vi "ALTS-2015 Confirm Test Selection DI.vi"(8 "error in":errorcluster, 11 "Station Cluster":T1) -> (0 "error out":errorcluster, 3 "Test Type Selection Successful":bool)   [LabVIEW 2013]
uses:
  Controls/ALTS-2015 Station Cluster.ctl
  Controls/ALTS-2015 LV2GBL Station Info Options.ctl
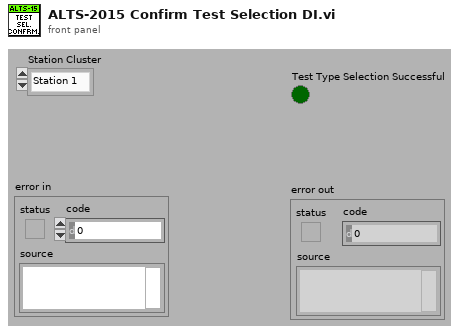
[diagram p1: front panel]
types:
  T1 = typedef "ALTS-2015 Station Cluster.ctl" = enum16{"Station 1", "Station 2", "Station 3", "Station 4"}
  T2 = typedef "ALTS-2015 LV2GBL Station Info Options.ctl" = enum16{"Init", "Read", "Read All", "Write Sensor ID", "Write  Work Order", "Write Serial Number", "Write Test Data", "Write Station Status", "Write Station Occupancy", "Write Station Test Type", "Write Rerun", "Write Load Decision", "Write Robot Action", "Clear All", "Clear Test Result"}
  T3 = typedef "ALTS-2015 Station Details.ctl" = cluster{"Station Number":string, "Work Order Number":string, "Sensor Name":string, "Pressure (PSI)":string, "Flow (SCCM)":string, "Test Time ":string, "Test Result":string, "Serial Number":string, "Station Status":T4, "SW assigned UUT":bool, "Rerun Count":i32, "Test Type":i32, "Load Decision":i32, "Robot Action":T5}
  T4 = typedef "ALTS-2015 Status Ring Indicator.ctl" = u16
  T5 = typedef "ALTS-2015 Robot Actions.ctl" = enum16{"Loading...", "Unloading...", "Reruning...", "No Action"}
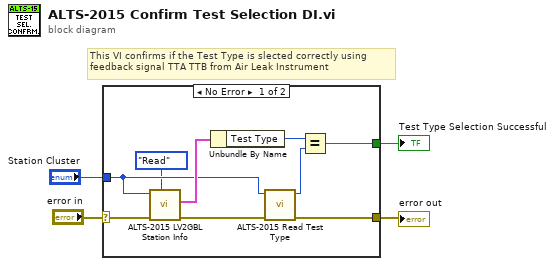
[diagram p0: block diagram]
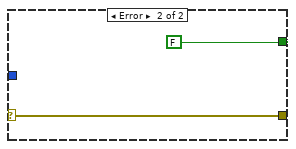
[diagram p2: hidden frame]
diagram:
  # "This VI confirms if the Test Type is slected correctly using \nfeedback signal TTA TTB from Air Leak Instrument"
  n1 = case shown="No Error" "error in" {
    selector: "error in" -> [w13 w15]
    tunnel: [w12 w15] -> w4
    tunnel: "Station Cluster" -> [w9 _]
    tunnel: [w7 FALSE] -> w1
    frame No Error {
      n2 = call "ALTS-2015 LV2GBL Station Info.vi"("Options"=ALTS-2015_LV2GBL_Station_Info_Options."Read", "error in"=w13, "Station Cluster"=w9) -> ("error out"=w11:errorcluster, "Station Details"=w10:T3)  [unwired: 6 in, 1 out]
      n3 = Unbundle By Name(w10) -> ("Test Type"=w8:i32)
      n4 = call "ALTS-2015 Read Test Type.vi"("error in"=w11, "Station Cluster"=w9) -> ("error out"=w12:errorcluster, "Test Type"=w6:i32)  [unwired: 8 in]
      n5 = Equal?(x=w8, y=w6) -> (x = y?=w7:bool)
    }
    frame Error {
    }
  }
  "error out" <- w4
  "Test Type Selection Successful" <- w1
